vi "ABR-Adapt Number of Averages.vi"(0 "Runtime":T1, 5 "Amplitude":dbl, 11 "error in (no error)":errorcluster) -> (4 "Runtime out":T1, 15 "error out":errorcluster)   [LabVIEW 2020]
uses:
  Typedefs/ABR-Runtime Data.ctl
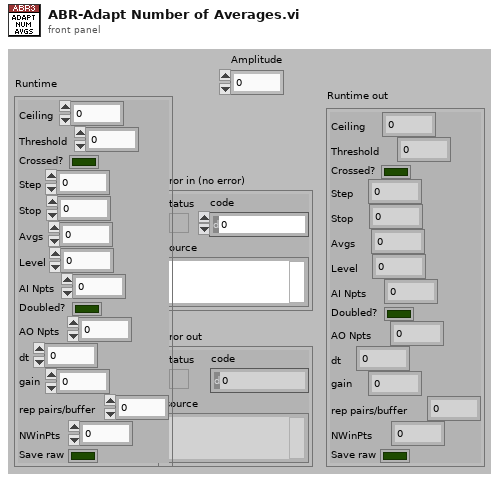
[diagram p1: front panel]
types:
  T1 = typedef "ABR-Runtime Data.ctl" = cluster{"Ceiling":dbl, "Threshold":dbl, "Crossed?":bool, "Step":dbl, "Stop":i32, "Avgs":i32, "Level":dbl, "AI Npts":i32, "Doubled?":bool, "AO Npts":i32, "dt":dbl, "gain":dbl, "rep pairs/buffer":i32, "NWinPts":i32, "Save raw":bool}
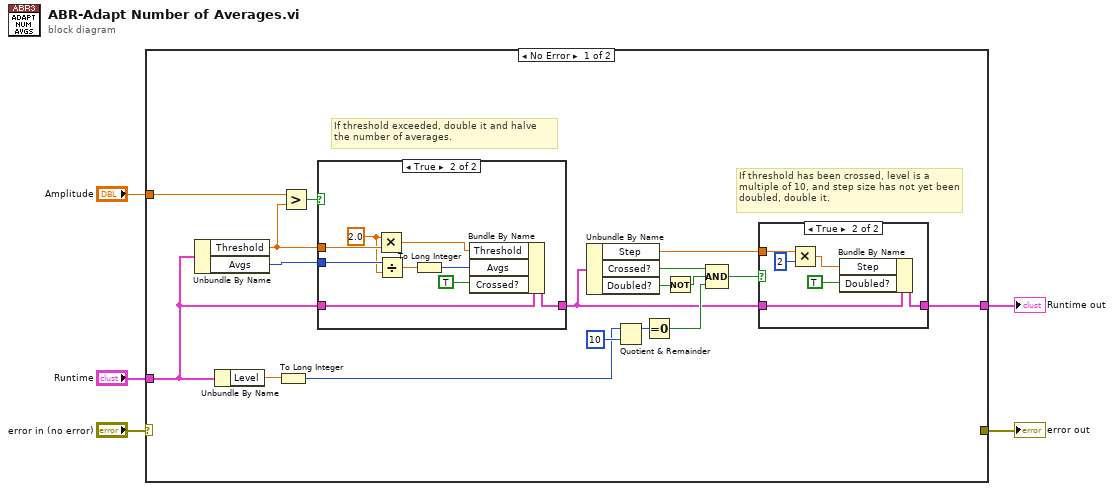
[diagram p0: block diagram]
diagram:
  n1 = case shown="No Error" "error in (no error)" {
    selector: "error in (no error)" -> [_ w40]
    tunnel: "Runtime" -> [w20 w41]
    tunnel: "Amplitude" -> [w22 _]
    tunnel: [w21 w41] -> w2
    tunnel: [_ w40] -> w1
    frame No Error {
      # "If threshold has been crossed, level is a multiple of 10, and step size has not yet been doubled, double it."
      # "If threshold exceeded, double it and halve the number of averages."
      n2 = Unbundle By Name(w20) -> ("Threshold"=w17:dbl, "Avgs"=w16:i32)
      n3 = Unbundle By Name(w20) -> ("Level"=w15:dbl)
      n4 = To Long Integer(number=w15) -> (32bit integer=w13:i32)
      n5 = Greater?(x=w22, y=w17) -> (0:w14:bool)
      n6 = case shown="True" w14 {
        tunnel: w20 -> [w30 w32]
        tunnel: w17 -> [_ w39]
        tunnel: w16 -> [_ w38]
        tunnel: [w30 w34] -> w6
        frame False {
        }
        frame True {
          w37 = 2.0 ("y")
          n7 = Multiply(x=w37, y=w39) -> (x*y=w36:dbl)
          n8 = Divide(x=w38, y=w37) -> (x/y=w35:dbl)
          n9 = To Long Integer(number=w35) -> (32bit integer=w33:i32)
          n10 = Bundle By Name(cluster=w32, "Threshold"=w36, "Avgs"=w33, "Crossed?"=TRUE) -> (w34:T1)
        }
      }
      n11 = Unbundle By Name(w6) -> ("Step"=w7:dbl, "Crossed?"=w11:bool, "Doubled?"=w12:bool)
      n12 = Quotient & Remainder(x=w13, y=10) -> (x-y*floor(x/y)=w18:i32)  [unwired: 1 out]
      n13 = Equal To 0?(x=w18) -> (x = 0?=w9:bool)
      n14 = Not(x=w12) -> (.not. x?=w10:bool)
      n15 = Compound Arithmetic op=AND(w11, w10, w9) -> (w8:bool)
      n16 = case shown="True" w8 {
        tunnel: [w23 w26] -> w21
        tunnel: w7 -> [_ w25]
        tunnel: w6 -> [w23 w24]
        frame False {
        }
        frame True {
          n17 = Multiply(x=w25, y=2) -> (x*y=w28:dbl)
          n18 = Bundle By Name(cluster=w24, "Step"=w28, "Doubled?"=TRUE ("Crossed?")) -> (w26:T1)
        }
      }
    }
    frame Error {
    }
  }
  "error out" <- w1
  "Runtime out" <- w2
